vi "trimOffLastChar.vi"(11 "String in":string) -> (3 "String out":string)   [LabVIEW 2013]
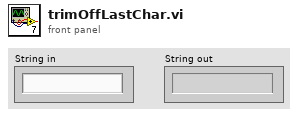
[diagram p1: front panel]
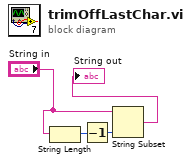
[diagram p0: block diagram]
diagram:
  n1 = String Length(string="String in") -> (length=w2:i32)
  n2 = Decrement(x=w2) -> (x-1=w1:i32)
  n3 = String Subset(string="String in", length (rest)=w1) -> (substring=→"String out":string)  [unwired: 1 in]
